vi "PID.vi"() -> ()   [LabVIEW 2021]
panel:
  out "output":dbl
  in  "input":dbl
  in  "reference":dbl
  in  "PID gains":cluster{"Kp":dbl, "Ki":dbl, "Kd":dbl}={"Kp"=1.0, "Ki"=0.1, "Kd"=0.0}
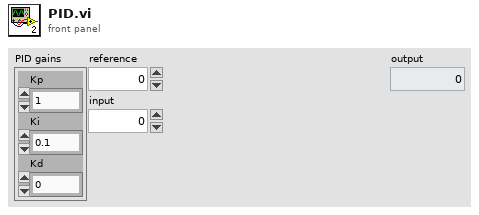
[diagram p1: front panel]
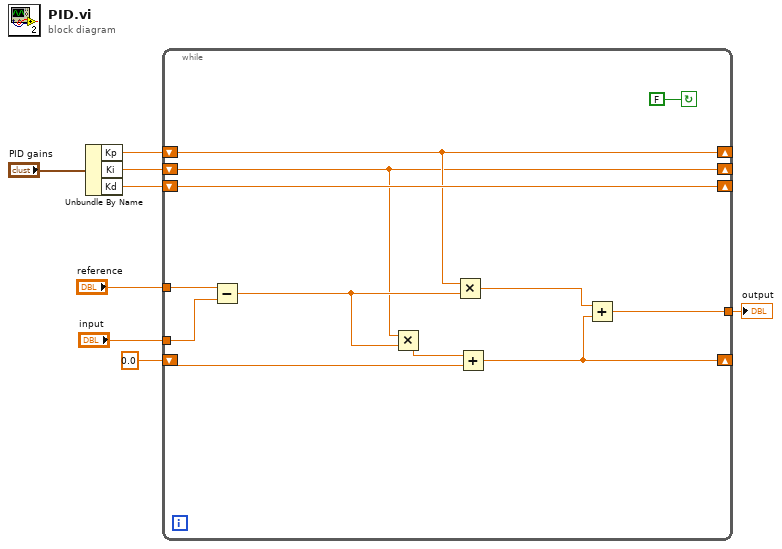
[diagram p0: block diagram]
diagram:
  n1 = Unbundle By Name("PID gains") -> ("Kp"=w7:dbl, "Ki"=w6:dbl, "Kd"=w5:dbl)
  n2 = while {
    shift-right: [w16] -> _
    shift-left: w7 -> [w16]
    shift-right: [w9] -> _
    shift-left: w6 -> [w9]
    shift-right: [w20] -> _
    shift-left: w5 -> [w20]
    tunnel: "reference" -> [w18]
    tunnel: "input" -> [w17]
    tunnel: [w14] -> w2
    shift-right: [w13] -> _
    shift-left: 0.0 ("input") -> [w12]
    stop <- FALSE continue-if-true
    n3 = Subtract(x=w18, y=w17) -> (x-y=w10:dbl)
    n4 = Multiply(x=w9, y=w10) -> (x*y=w11:dbl)
    n5 = Multiply(x=w16, y=w10) -> (x*y=w15:dbl)
    n6 = Add(x=w11, y=w12) -> (x+y=w13:dbl)
    n7 = Add(x=w15, y=w13) -> (x+y=w14:dbl)
  }
  "output" <- w2
